vi "Change Controls.vi"(7 "Adjust All?":bool=TRUE, 8 "Indicators":string[][](array[string]), 9 "Controls":string[][](array[string]), 10 "VI Index":i32, 11 "VI Data":T1[](array[typedef])) -> (3 "VI Data out":T1[](array[typedef]))   [LabVIEW 2023, in "VI Properties Editor.lvlib"]
uses:
  VI Properties Editor.lvlib
  Cluster Data.ctl
  <vilib>/picture/picture.llb/imagedata.ctl
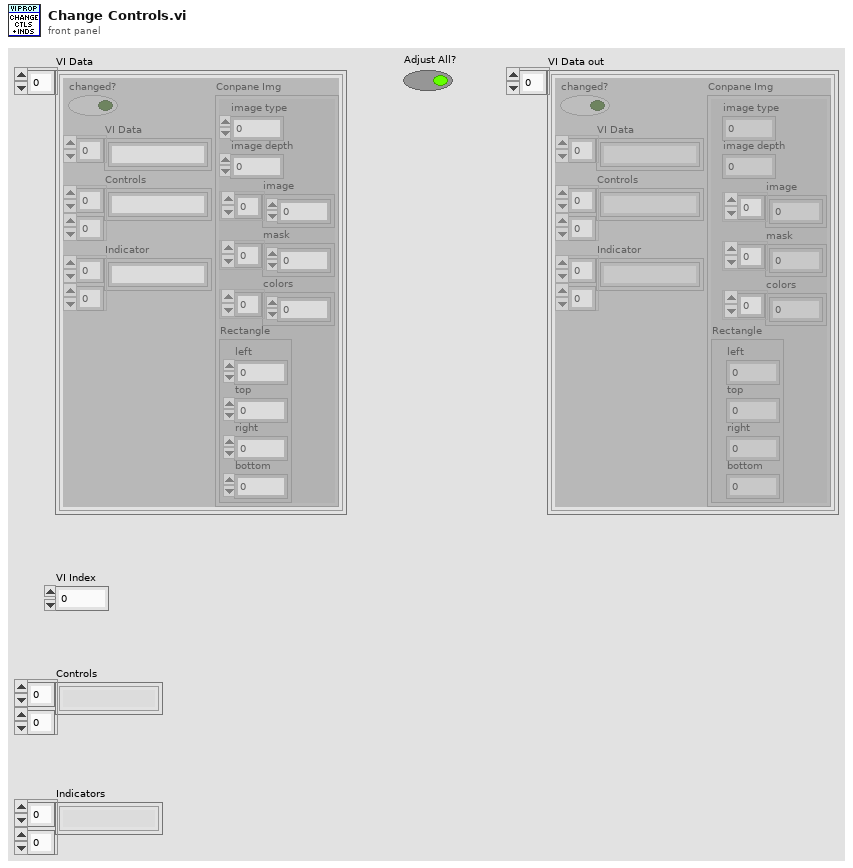
[diagram p1: front panel]
types:
  T1 = typedef "VI Properties Editor.lvlib/Cluster Data.ctl" = cluster{"changed?":bool, "VI Data":string[], "Controls":string[][], "Indicator":string[][], "Conpane Img":T2}
  T2 = typedef "imagedata.ctl" = cluster{"image type":i32, "image depth":i32, "image":u8[], "mask":u8[], "colors":u32[], "Rectangle":cluster{"left":i16, "top":i16, "right":i16, "bottom":i16}}
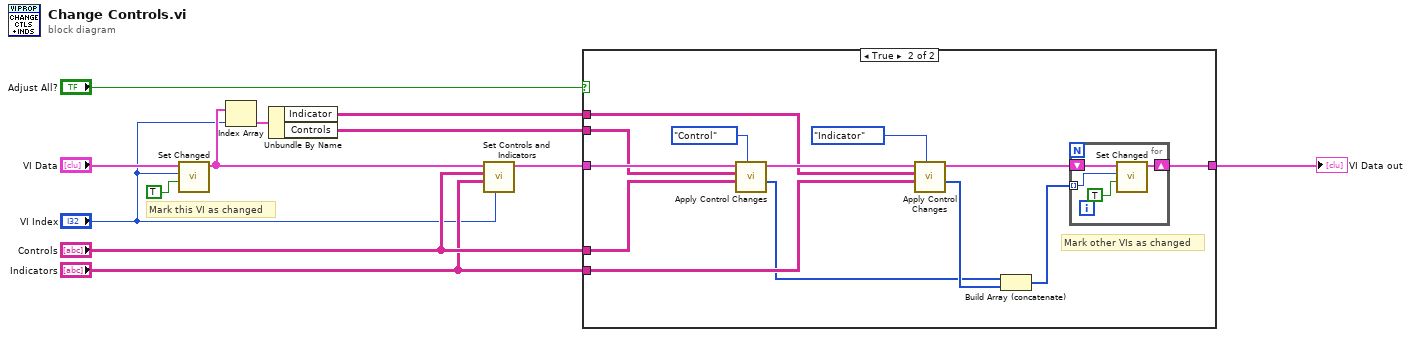
[diagram p0: block diagram]
diagram:
  # "Mark this VI as changed"
  n1 = call "Set Changed.vi"("changed?"=TRUE, "VI Index"="VI Index", "Array in"="VI Data") -> ("Array out"=w8:T1[])  [unwired: 8 in]
  n2 = Index Array(array=w8, index="VI Index") -> (element=w12:T1)
  n3 = Unbundle By Name(w12) -> ("Indicator"=w9:string[][], "Controls"=w2:string[][])
  n4 = call "Set Controls and Indicators.vi"("VI Index"="VI Index", "Indicators"="Indicators", "Controls"="Controls", "Data In"=w8) -> ("Data Out"=w11:T1[])  [unwired: 7 in]
  n5 = case shown="True" "Adjust All?" {
    tunnel: "Controls" -> [_ w23]
    tunnel: w2 -> [_ w24]
    tunnel: w9 -> [_ w22]
    tunnel: "Indicators" -> [_ w21]
    tunnel: w11 -> [w13 w26]
    tunnel: [w13 w19] -> w4
    frame False {
    }
    frame True {
      # "Mark other VIs as changed"
      n6 = call "Apply Control Changes.vi"("Type"=enum16{"Control", "Indicator"}."Control", "new"=w23, "old"=w24, "Data In"=w26) -> ("Changed indices"=w14:i32[], "Data Out"=w25:T1[])  [unwired: 6 in]
      n7 = call "Apply Control Changes.vi"("Type"=enum16{"Control", "Indicator"}."Indicator", "new"=w21, "old"=w22, "Data In"=w25) -> ("Changed indices"=w20:i32[], "Data Out"=w17:T1[])  [unwired: 6 in]
      n8 = Build Array (concatenate)(w14, w20) -> (w18:i32[])
      n9 = for {
        shift-right: [w29] -> w19
        shift-left: w17 -> [w30]
        tunnel: w18 -> [w28] mode=indexing
        n10 = call "Set Changed.vi"("changed?"=TRUE ("new element/subarray"), "VI Index"=w28, "Array in"=w30) -> ("Array out"=w29:T1[])  [unwired: 8 in]
      }
    }
  }
  "VI Data out" <- w4
